vi "dummy steering.vi"() -> ()   [LabVIEW 2012]
uses:
  <vilib>/Analysis/1siggen.llb/Ramp Pattern by Samples.vi
  <vilib>/gmath/statdist.llb/Normal PDF.vi
  <vilib>/gmath/NI_Gmath.lvlib
  <vilib>/Analysis/NI_AALBase.lvlib
panel:
  in  "Velocity\nGain":dbl
  out "Desired Velocity":i32
  out "Desired Heading":i32
  out "size(s)":i32
  out "Array":dbl[](array[numeric])
  out "Waveform Graph":dbl[](graph)
  in  "NewSteerAngle":dbl
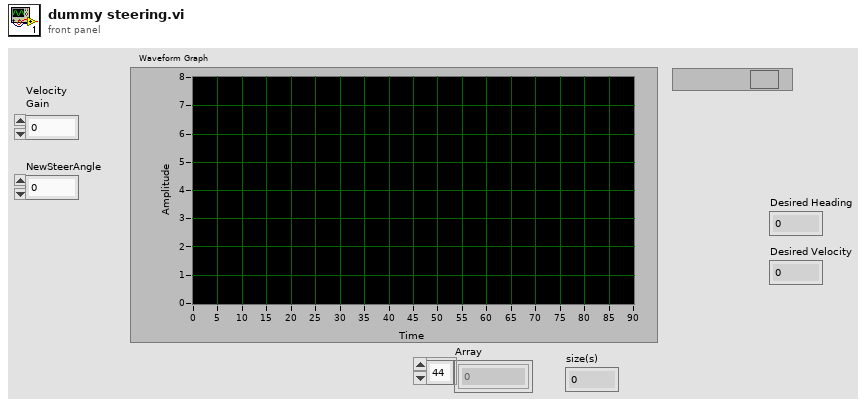
[diagram p1: front panel]
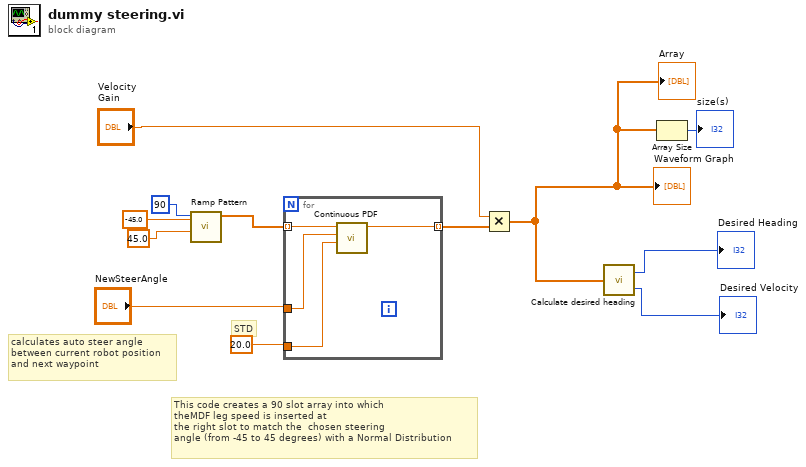
[diagram p0: block diagram]
diagram:
  # "calculates auto steer angle\nbetween current robot position\nand next waypoint"
  # "STD"
  # "This code creates a 90 slot array into which\ntheMDF leg speed is inserted at\nthe right slot to match the  chosen steering\nangle (from -45 to 45 degrees) with a Normal Distribution"
  n1 = call-poly <vilib>:"Ramp Pattern.vi"("start"=45.0, "end"=-45.0 ("end (Normal)"), "samples"=90) -> ("Ramp Pattern"=w10:dbl[])  [unwired: 7 in, 1 out]
  n2 = for {
    tunnel: w10 -> [w16] mode=indexing
    tunnel: 20.0 ("std (Normal)") -> [w15]
    tunnel: [w14] -> w3 mode=indexing
    tunnel: "NewSteerAngle" -> [w13]
    n3 = call-poly <vilib>:"Continuous PDF.vi"("std"=w15, "mean"=w13, "x"=w16) -> ("pdf(x)"=w14:dbl)  [unwired: 7 in, 1 out]
  }
  n4 = Multiply(x="Velocity\nGain", y=w3) -> (x*y=w1:dbl[])
  "Waveform Graph" <- w1
  "Array" <- w1
  n5 = call "Calculate desired heading.vi"("Arbiter Array"=w1) -> ("Desired Heading"=→"Desired Heading":i32, "Desired Velocity"=→"Desired Velocity":i32)
  n6 = Array Size(array=w1) -> (size(s)=→"size(s)":i32)
